vi "Do.vi"(8 "error in (no error)":errorcluster, 10 "In Range":T1, 11 "Rule In":refnum<class "Rule.lvclass">) -> (0 "error out":errorcluster, 1 "Out Range":T1[](array[typedef]), 2 "Label":string[](array[string]), 3 "Rule Out":refnum<class "Rule.lvclass">)   [LabVIEW 2021, in "Rule.lvclass"]
uses:
  Rule.lvclass
  xmas.ctl
  Rule.lvclass/Rule.ctl
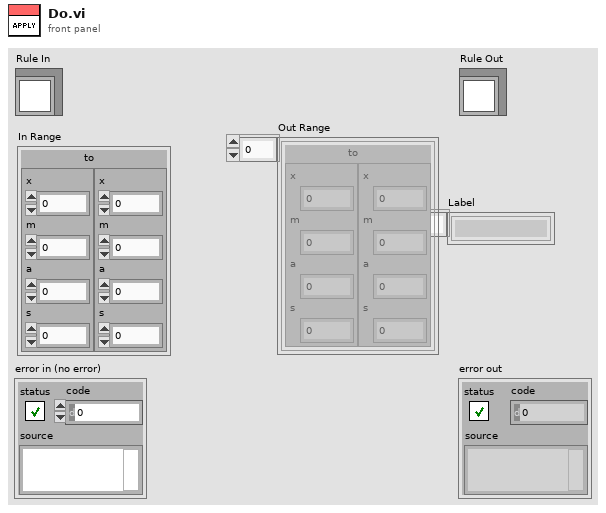
[diagram p1: front panel]
types:
  T1 = typedef "xmas.ctl" = cluster{"from":cluster{"x":u64, "m":u64, "a":u64, "s":u64}, "to":cluster{"x":u64, "m":u64, "a":u64, "s":u64}}
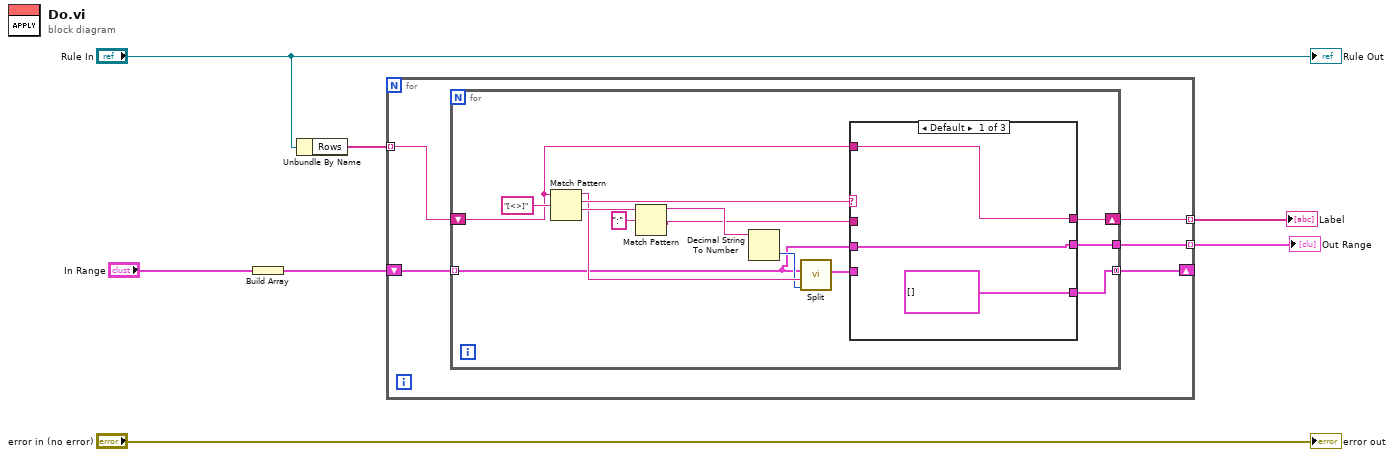
[diagram p0: block diagram]
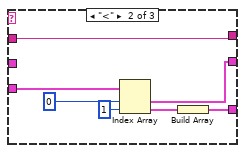
[diagram p2: hidden frame]
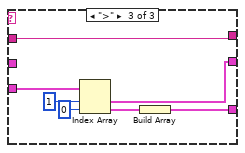
[diagram p3: hidden frame]
diagram:
  n1 = Build Array("In Range") -> (w1:T1[])
  n2 = Unbundle By Name("Rule In") -> ("Rows"=w6:string[])
  n3 = for {
    tunnel: w6 -> [w11] mode=indexing
    tunnel: [w12] -> w3 mode=indexing
    tunnel: [w9] -> w4 mode=indexing
    shift-right: [w8] -> _
    shift-left: w1 -> [w10]
    n4 = for {
      tunnel: w10 -> [w13] mode=indexing
      tunnel: [w15] -> w9
      shift-right: [w21] -> w12
      shift-left: w11 -> [w20]
      tunnel: [w14] -> w8 mode=concatenating
      n5 = Match Pattern(string=w20, regular expression="[<>]") -> (before substring=w18:string, match substring=w25:string, after substring=w24:string)  [unwired: 1 in, 1 out]
      n6 = Match Pattern(string=w24, regular expression=":") -> (before substring=w22:string, after substring=w19:string)  [unwired: 1 in, 2 out]
      n7 = Decimal String To Number(string=w22) -> (number=w17:i32)  [unwired: 2 in, 1 out]
      n8 = call "Split.vi"("Val"=w17, "Label"=w18, "Cluster"=w13) -> ("Result"=w16:T1[])  [unwired: 8 in]
      n9 = case shown="Default" w25 {
        tunnel: [w29 w36 w43] -> w21
        tunnel: w20 -> [w29 _ _]
        tunnel: w19 -> [_ w36 w43]
        tunnel: w16 -> [_ w35 w42]
        tunnel: [w27 w33 w40] -> w15
        tunnel: [T1[] [] ("Cluster") w30 w37] -> w14
        tunnel: w13 -> [w27 _ _]
        frame Default {
        }
        frame "<" {
          n10 = Index Array(array=w35, index #1=0 ("index"), index #2=1 ("index")) -> (element #1=w33:T1, element #2=w31:T1)
          n11 = Build Array(w31) -> (w30:T1[])
        }
        frame ">" {
          n12 = Index Array(array=w42, index #1=1 ("index"), index #2=0 ("index")) -> (element #1=w40:T1, element #2=w38:T1)
          n13 = Build Array(w38) -> (w37:T1[])
        }
      }
    }
  }
  "Label" <- w3
  "Out Range" <- w4
  "error out" <- "error in (no error)"
  "Rule Out" <- "Rule In"
